vi "布尔非转非法数字.vi"(1 "布尔数组":bool[](array[boolean])) -> (0 "NaN":dbl[](array[numeric]))   [LabVIEW 2021]
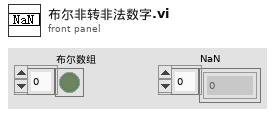
[diagram p1: front panel]
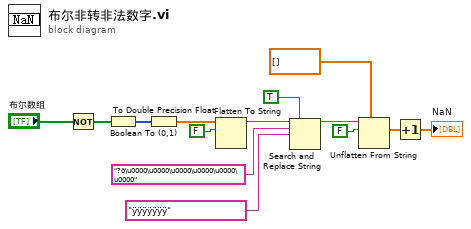
[diagram p0: block diagram]
diagram:
  n1 = Not(x="布尔数组") -> (.not. x?=w1:bool[])
  n2 = Boolean To (0,1)(Boolean=w1) -> (0, 1=w3:i16[])
  n3 = To Double Precision Float(number=w3) -> (double precision float=w4:dbl[])
  n4 = Flatten To String(anything=w4, prepend array or string size? (T)=FALSE ("预置数组或字符串大小？ (T)")) -> (data string=w6:string)  [unwired: 2 in, 2 out]
  n5 = Search and Replace String(replace all?=TRUE ("替换全部？(F)"), input string=w6, search string="?ð\u0000\u0000\u0000\u0000\u0000\u0000", replace string="ÿÿÿÿÿÿÿ" ("替换字符串(\"\")")) -> (result string=w10:string)  [unwired: 4 in, 3 out]
  n6 = Unflatten From String(type=dbl[] [] ("值"), binary string=w10, data includes array or string size? (T)=FALSE ("数据中包含数组或字符串大小？(T)")) -> (value=w11:dbl[])  [unwired: 2 in, 2 out]
  n7 = Increment(x=w11) -> (x+1=→"NaN":dbl[])
